vi "Set SMU1 Current Level.vi"(10 "R":i32) -> (2 "Smu1 current":dbl)   [LabVIEW 2010]
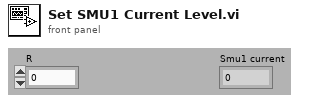
[diagram p1: front panel]
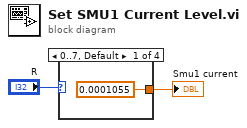
[diagram p0: block diagram]
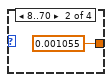
[diagram p2: hidden frame]
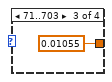
[diagram p3: hidden frame]
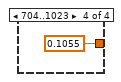
[diagram p4: hidden frame]
diagram:
  n1 = case shown="0..7, Default" "R" {
    tunnel: [0.0001055 ("R 2") 0.001055 ("R 2") 0.01055 ("R 2") 0.1055 ("R 2")] -> w1
    frame 0..7, Default {
    }
    frame 8..70 {
    }
    frame 71..703 {
    }
    frame 704..1023 {
    }
  }
  "Smu1 current" <- w1
